vi "Panel (sub vi).vi"(9 "Record":string[][](array[string])=[["Name", "Points", "Time", "Win / Lose"]]) -> (0 "EXIT 2":bool, 1 "Record":string[][](array[string])=[["Name", "Points", "Time", "Win / Lose"]], 2 "PLAY 2":bool)   [LabVIEW 2014]
uses:
  READY.ctl
panel:
  in  "EXIT":bool
  in  "PLAY":T1
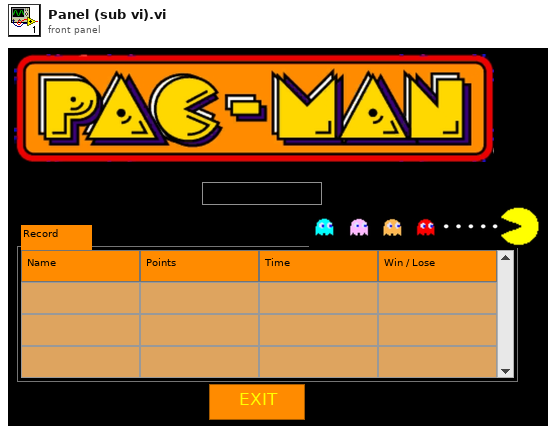
[diagram p1: front panel]
types:
  T1 = typedef "READY.ctl" = bool
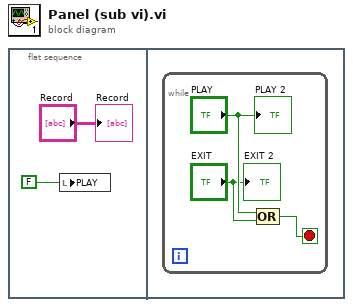
[diagram p0: block diagram]
diagram:
  n1 = flat-sequence {
    frame #0 {
      n2 = local write "PLAY"(FALSE ("OK Button")) -> ()
      "Record" <- "Record"
    }
    frame #1 {
      n3 = while {
        stop <- w3 stop-if-true
        n4 = Compound Arithmetic op=OR("PLAY", "EXIT") -> (w3:T1)
        "PLAY 2" <- "PLAY"
        "EXIT 2" <- "EXIT"
      }
    }
  }
